vi "3A Helper - DegreetoPWM.vi"(9 "Rudder Angle":T1, 10 "Rudder Trim":dbl(slide) scale=-20.0..20.0, 11 "Rudder Range (deg)":dbl=100.0) -> (3 "Servo Position (us)":u32)   [LabVIEW 2011]
uses:
  2-Think/2 Typedefs/rudder angle.ctl
panel:
  in  "PWM center point":dbl=1620.0
  in  "PWM microseconds\nper degree":dbl=-8.8
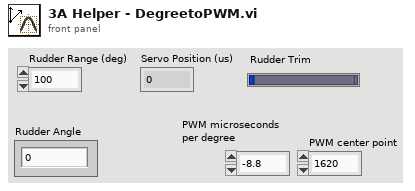
[diagram p1: front panel]
types:
  T1 = typedef "rudder angle.ctl" = dbl
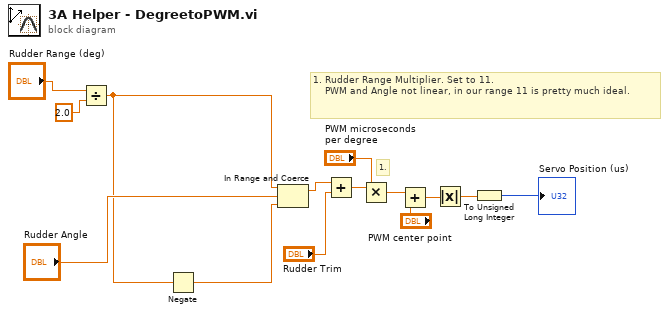
[diagram p0: block diagram]
diagram:
  # "1."
  # "1. Rudder Range Multiplier. Set to 11.\n    PWM and Angle not linear, in our range 11 is pretty much ideal."
  n1 = Divide(x="Rudder Range (deg)", y=2.0) -> (x/y=w2:dbl)
  n2 = Negate(x=w2) -> (-x=w3:dbl)
  n3 = In Range and Coerce(upper limit=w2, x="Rudder Angle", lower limit=w3) -> (coerced(x)=w7:T1)  [unwired: 1 out]
  n4 = Add(x=w7, y="Rudder Trim") -> (x+y=w8:T1)
  n5 = Multiply(x=w8, y="PWM microseconds\nper degree") -> (x*y=w10:T1)
  n6 = Add(x=w10, y="PWM center point") -> (x+y=w12:T1)
  n7 = Absolute Value(x=w12) -> (abs(x)=w13:T1)
  n8 = To Unsigned Long Integer(number=w13) -> (unsigned 32bit integer=→"Servo Position (us)":u32)
